vi "start.vi"(8 "error in (no error)":errorcluster, 11 "k3390_AWG in":refnum<class "k3390_AWG.lvclass">) -> (0 "error out":errorcluster, 3 "k3390_AWG out":refnum<class "k3390_AWG.lvclass">)   [LabVIEW 2009, in "Hardware.lvlib" / "Channels.lvlib" / "k3390_AWG.lvclass"]
uses:
  k3390_AWG.lvclass
  k3390_AWG.lvclass/k3390_AWG.ctl
  <instrlib>/Keithley 3390/Keithley 3390.lvlib
  Generic/DDSOutput.lvclass
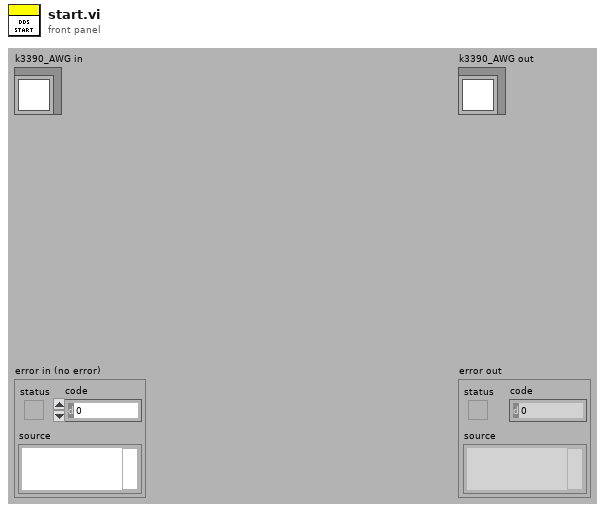
[diagram p1: front panel]
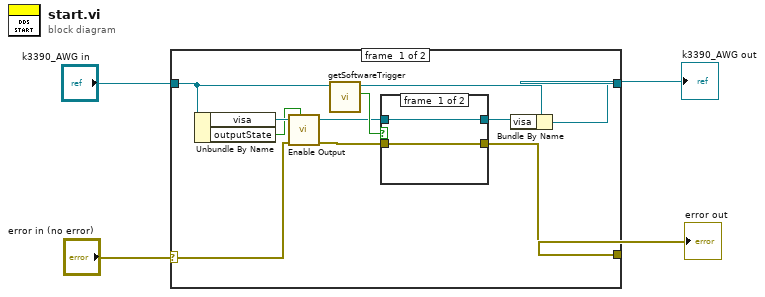
[diagram p0: block diagram]
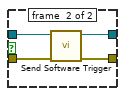
[diagram p2: hidden frame]
diagram:
  n1 = case shown="No Error" "error in (no error)" {
    selector: "error in (no error)" -> [w15 w22]
    tunnel: "k3390_AWG in" -> [w13 w23]
    tunnel: [w14 w23] -> w2
    tunnel: [w12 w22] -> w1
    frame #0 {
      n2 = Unbundle By Name(w13) -> ("visa"=w11:refnum<visa-resource-name>, "outputState"=w5:bool)
      n3 = call <instrlib>:"Enable Output.vi"("Enable Output (T: Enable)"=w5, "error in (no error)"=w15, "VISA resource name"=w11) -> ("error out"=w6:errorcluster, "VISA resource name out"=w8:refnum<visa-resource-name>)  [unwired: 7 in]
      n4 = call "getSoftwareTrigger.vi"("DDSOutput in"=w13) -> ("softwareTrigger"=w9:bool, "DDSOutput out"=w10:refnum<class "k3390_AWG.lvclass">)  [unwired: 8 in, 1 out]
      n5 = case shown="False" w9 {
        tunnel: w8 -> [w17 w21]
        tunnel: [w17 w20] -> w7
        tunnel: w6 -> [w16 w19]
        tunnel: [w16 w18] -> w12
        frame #0 {
        }
        frame #1 {
          n6 = call <instrlib>:"Send Software Trigger.vi"("error in (no error)"=w19, "VISA resource name"=w21) -> ("error out"=w18:errorcluster, "VISA resource name out"=w20:refnum<visa-resource-name>)  [unwired: 8 in]
        }
      }
      n7 = Bundle By Name(cluster=w10, "visa"=w7) -> (w14:refnum<class "k3390_AWG.lvclass">)
    }
    frame #1 {
    }
  }
  "error out" <- w1
  "k3390_AWG out" <- w2
